vi "Create Alarm State Update User Event.vi"(8 "error in (no error)":errorcluster) -> (0 "error out":errorcluster, 3 "Alarm State":refnum<user-event>)   [LabVIEW 2015, in "Alarm Handler Actor.lvclass"]
uses:
  Alarm Handler Actor.lvclass
  State.ctl
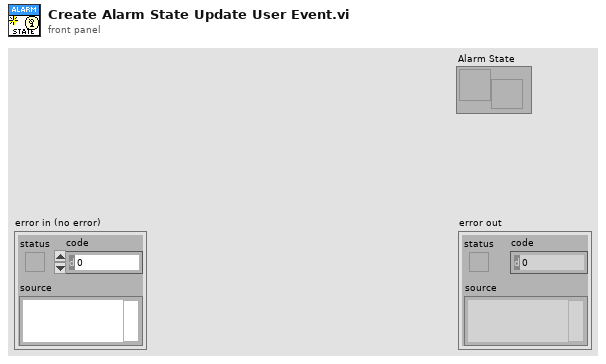
[diagram p1: front panel]
types:
  T1 = typedef "Alarm Handler Actor.lvclass/State.ctl" = cluster{"Alarms":cluster{"Alarm Number":i32}[]}
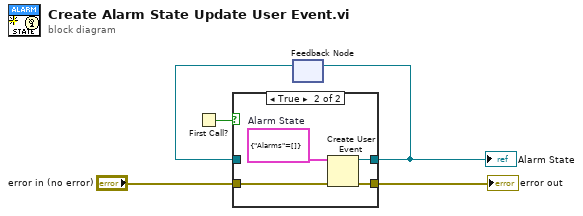
[diagram p0: block diagram]
diagram:
  n1 = First Call?() -> (First Call?: T/F=w3:bool)
  n2 = feedback #1() -> (w2:refnum<user-event>)  [unwired: 1 in]
  n3 = case shown="True" w3 {
    tunnel: "error in (no error)" -> [w6 w11]
    tunnel: [w6 w10] -> w4
    tunnel: [w7 w9] -> w1
    tunnel: w2 -> [w7 _]
    frame False {
    }
    frame True {
      w8 = T1 {"Alarms"=[]}  # Alarm State
      n4 = Create User Event(user event datatype=w8, error in=w11) -> (user event=w9:refnum<user-event>, error out=w10:errorcluster)
    }
  }
  "error out" <- w4
  "Alarm State" <- w1
  n5 = feedback-in #1(w1) -> ()
